vi "Rotary mm_s to rpm conversion.vi"(8 "error in (no error)":errorcluster, 9 "Enter the Final Velocity (m/s) 3":dbl=1.0 min=0.001 max=2.0 step=0.001 format="%.3f", 10 "Wear Track Diameter":dbl=1.0 min=0.001 max=4.0 step=0.001 format="%.3f", 11 "Enter initial Velocity (m/s)  3":dbl=2.0 min=0.001 max=2.0 step=0.001 format="%.3f") -> (0 "error out":errorcluster, 2 "Final Speed (RPM) 3":dbl=1.0 min=0.1 max=3000.0 step=0.1 format="%.1f", 3 "Initial Speed (RPM) 2":dbl=100.0 min=0.1 max=3000.0 step=0.1 format="%.1f")   [LabVIEW 2025]
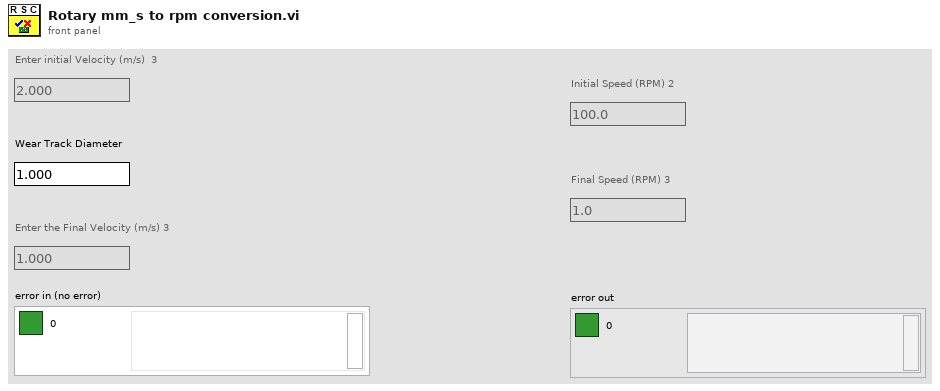
[diagram p1: front panel]
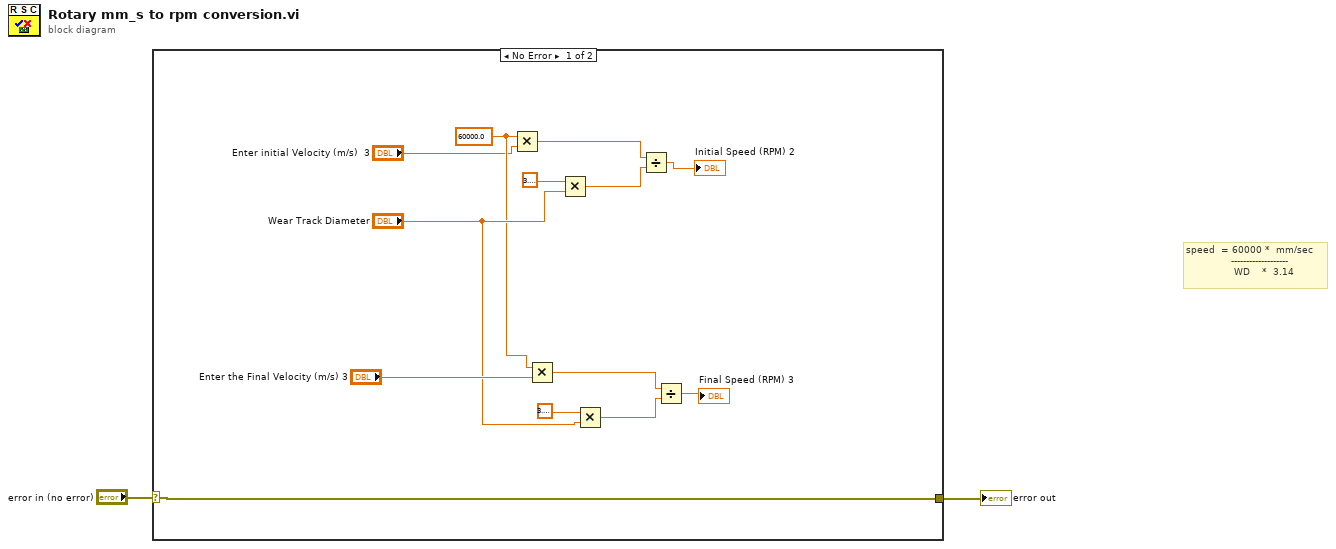
[diagram p0: block diagram]
diagram:
  # "speed  = 60000 *  mm/sec\n               -------------------\n                WD    *  3.14"
  n1 = case shown="No Error" "error in (no error)" {
    selector: "error in (no error)" -> [w3 _]
    tunnel: [w3 _] -> w2
    frame No Error {
      w11 = 60000.0 ("x")
      n2 = Multiply(x=w11, y="Enter initial Velocity (m/s)  3") -> (x*y=w7:dbl)
      n3 = Multiply(x=w11, y="Enter the Final Velocity (m/s) 3") -> (x*y=w8:dbl)
      n4 = Multiply(x=3.141592653589793, y="Wear Track Diameter") -> (x*y=w6:dbl)
      n5 = Multiply(x=3.141592653589793, y="Wear Track Diameter") -> (x*y=w9:dbl)
      n6 = Divide(x=w7, y=w6) -> (x/y=→"Initial Speed (RPM) 2":dbl)
      n7 = Divide(x=w8, y=w9) -> (x/y=→"Final Speed (RPM) 3":dbl)
    }
    frame Error {
    }
  }
  "error out" <- w2
